vi "ROSServiceProvider.vi"(2 "Response":T2, 3 "ROS":T3={"topic port"=1236, "Node"="/labview", "topic"="/robot/head/command_head_nod", "type"="std_msgs/Bool", "node port"=7000, "error "={"status"=FALSE, "code"=0, "source"=""}, "Direction"=enum."Publisher", "Update (ms)"=1, "FIFO size"=1}) -> ()   [LabVIEW 2012]
doc: "Opens new ports for services, updates services with master, and closes services"
uses:
  Console/Servers/ServerSubs/MyState.ctl
  _ROSDefinition.vi
  MessageBuilding/std_msgs/subs/i16Scalar.vi
  MessageBuilding/std_msgs/subs/stringScalar.vi
  SubVIs/_ROSDirection.ctl
  SubVIs/_ROSControl.ctl
panel:
  out "Queue":string
  out "Master Reply":T1(array[cluster])
  out "response":string
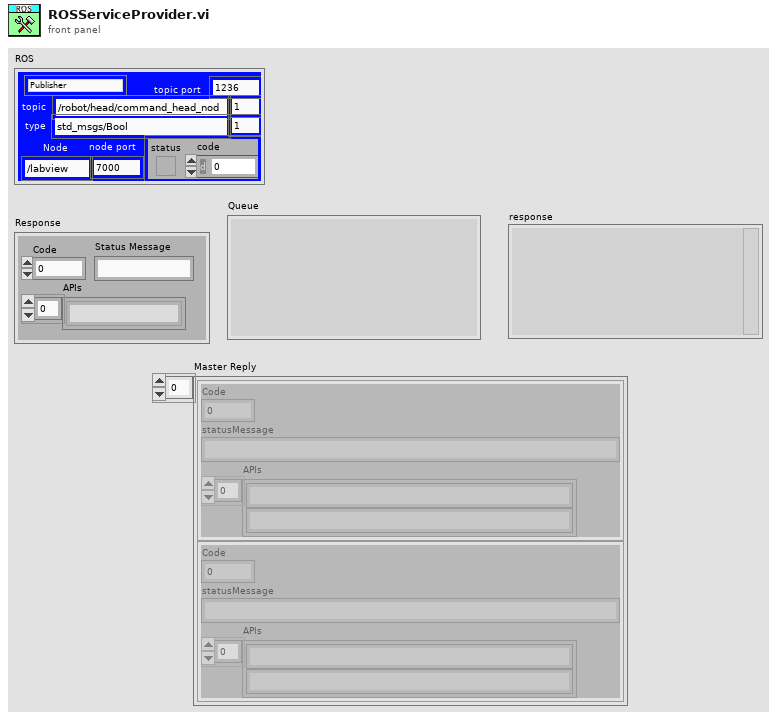
[diagram p1: front panel]
types:
  T1 = cluster{"Code":i8, "statusMessage":string, "APIs":string[]}[]
  T2 = cluster{"Code":i32, "Status Message":string, "APIs":string[]}
  T3 = typedef "_ROSControl.ctl" = cluster{"topic port":u16, "Node":string, "topic":string, "type":string, "node port":u16, "error ":errorcluster, "Direction":T4, "Update (ms)":u16, "FIFO size":u16}
  T4 = typedef "_ROSDirection.ctl" = enum16{"Node", "Publisher", "Subscriber", "ServiceClient", "ServiceProvider"}
  T5 = typedef "MyState.ctl" = enum16{"No Connection", "Registered", "Connected", "Close"}
  T6 = enum16{"Reset Log", "Add Client", "Remove Client", "Add Task"}
  T7 = typedef "ROSLog.ctl" = cluster{"Sent":string, "Reply":string, "MethodName":string, "success":bool, "Dir1":string, "Dir2":string, "Time Stamp":string, "error":errorcluster, "Preamble":string, "Midamble":string, "Postamble":string}
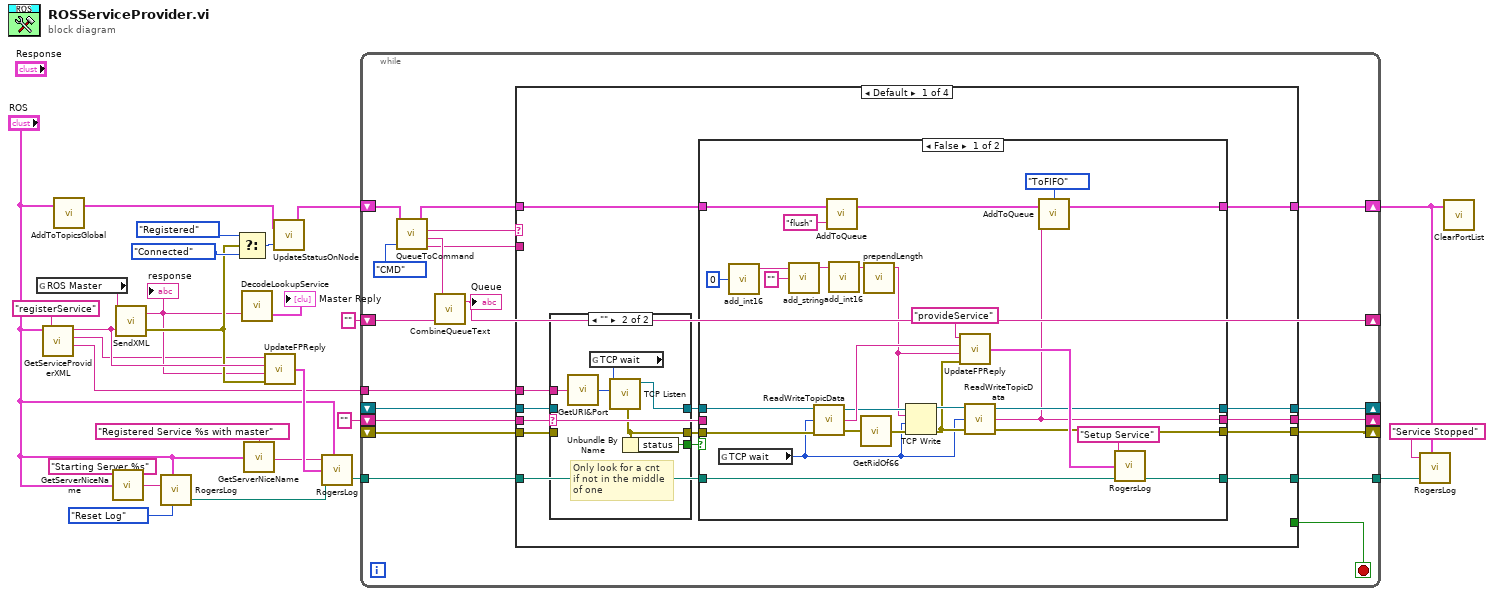
[diagram p0: block diagram]
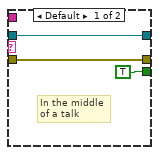
[diagram p2: hidden frame]
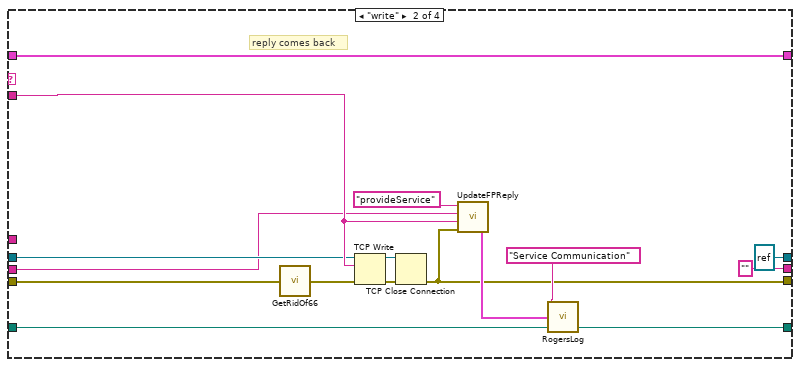
[diagram p4: hidden frame]
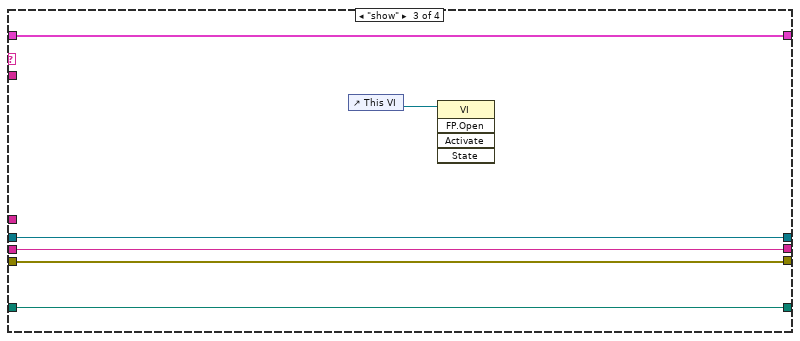
[diagram p5: hidden frame]
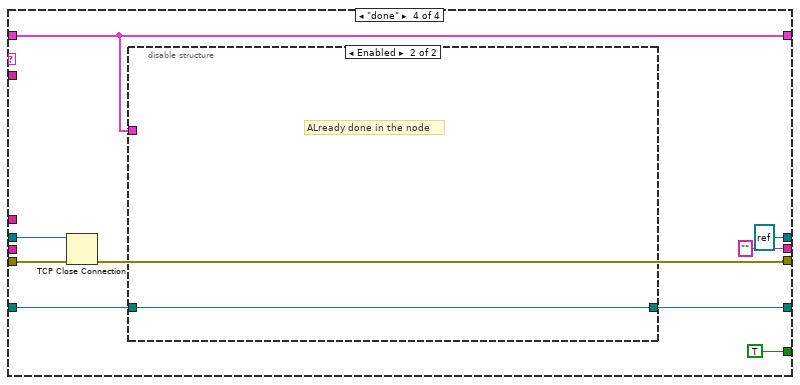
[diagram p6: hidden frame]
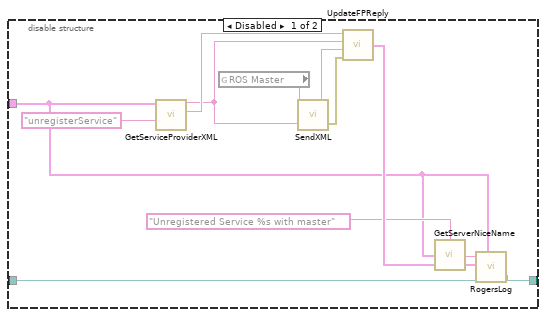
[diagram p7: hidden frame]
diagram:
  n1 = global read "_ROSDefinition.vi" "ROS Master"() -> (w23:string)
  n2 = call "GetServiceProviderXML.vi"("Method Name"="registerService", "ROS"="ROS") -> ("URI"=w6:string, "Method Name"=w9:string, "lookupService"=w24:string)  [unwired: 7 in]
  n3 = call "AddToTopicsGlobal.vi"("ROS in"="ROS") -> ("ROS out"=w3:T3)  [unwired: 2 in]
  n4 = call "GetServerNiceName.vi"("ROS"="ROS", "Text to add"="Starting Server %s") -> ("String"=w26:string)
  n5 = call "SendXML.vi"("Send"=w24, "URI in"=w23) -> ("error out"=w15:errorcluster, "Reply"=w14:string)
  "response" <- w14
  n6 = call "RogersLog.vi"("Text to add"=w26, "ROS"="ROS", "Task"=T6."Reset Log") -> ("LogPath out"=w18:path)  [unwired: 2 in, 1 out]
  n7 = Select(t=MyState."Registered" ("MyState"), s=w15, f=MyState."Connected" ("MyState")) -> (s? t:f=w20:T5)
  n8 = call "DecodeLookupService.vi"("Response"=w14) -> ("Reply"=→"Master Reply":T1)  [unwired: 2 in]
  n9 = call "GetServerNiceName.vi"("ROS"="ROS", "Text to add"="Registered Service %s with master") -> ("String"=w16:string)
  n10 = call "UpdateFPReply.vi"("error in (no error)"=w15, "Reply"=w14, "Sent"=w24, "method"=w9) -> ("Log"=w19:T7)
  n11 = call "UpdateStatusOnNode.vi"("MyState"=w20, "ROS"=w3) -> ("ROS out"=w2:T3)  [unwired: 1 in]
  n12 = call "RogersLog.vi"("Text to add"=w16, "ROS"="ROS", "Log"=w19, "LogPath in"=w18) -> ("LogPath out"=w11:path)  [unwired: 1 in, 1 out]
  n13 = while {
    tunnel: w11 -> [w46]
    tunnel: [w45] -> w10
    shift-right: [w41] -> _
    shift-left: "" ("New List") -> [w42]
    tunnel: w6 -> [w40]
    shift-right: [w35] -> _
    shift-left: _ -> [w32]
    shift-right: [w34] -> _
    shift-left: "" ("data out") -> [w30]
    shift-right: [w33] -> _
    shift-left: _ -> [w31]
    shift-right: [w28] -> w1
    shift-left: w2 -> [w39]
    stop <- w44 stop-if-true
    n14 = call "QueueToCommand.vi"("ROS"=w39, "Check"=enum16{"Cmd+FIFO", "FIFO", "CMD"}."CMD") -> ("ROS out"=w29:T3, "Command"=w37:string, "Queue log"=w43:string, "data"=w36:string)  [unwired: 1 in]
    n15 = call "CombineQueueText.vi"("Old List"=w42, "Queue In"=w43) -> ("New List"=w41:string)  [unwired: 1 in]
    "Queue" <- w41
    n16 = case shown="Default" w37 {
      tunnel: w29 -> [w59 w105 w123 w132]
      tunnel: w46 -> [w58 w108 w124 w131]
      tunnel: [w57 w107 w124 w130] -> w45
      tunnel: w36 -> [_ w113 _ _]
      tunnel: [w47 w105 w123 w132] -> w28
      tunnel: [_ _ _ TRUE] -> w44
      tunnel: w40 -> [w56 _ _ _]
      tunnel: [w55 refnum<k5> refnum ("connection ID out") w119 refnum<k5> refnum ("connection ID out")] -> w35
      tunnel: [w54 "" ("data out") w120 "" ("data out")] -> w34
      tunnel: [w53 w106 w121 w127] -> w33
      tunnel: w32 -> [w50 w111 w119 w128]
      tunnel: w31 -> [w51 w110 w121 w129]
      tunnel: w30 -> [w52 w109 w120 _]
      frame Default {
        n17 = case shown="\"\"" w52 {
          tunnel: [w63 w65] -> w49
          tunnel: [w62 w68] -> w60
          tunnel: w56 -> [_ w66]
          tunnel: w51 -> [w63 _]
          tunnel: w50 -> [w62 _]
          tunnel: [TRUE w64] -> w48
          frame Default {
            # "In the middle\nof a talk"
          }
          frame "" {
            # "Only look for a cnt\nif not in the middle\nof one"
            n18 = call "GetURI&Port.vi"("URI in"=w66) -> ("Port"=w69:u16)  [unwired: 1 out]
            n19 = global read "_ROSDefinition.vi" "TCP wait"() -> (w67:i32)
            n20 = call <vilib>:"TCP Listen.vi"("timeout ms (wait forever: -1)"=w67, "port"=w69) -> ("error out"=w65:errorcluster, "connection ID"=w68:refnum<k5>)  [unwired: 5 in, 3 out]
            n21 = Unbundle By Name(w65) -> ("status"=w64:bool)
          }
        }
        n22 = case shown="False" w48 {
          tunnel: w60 -> [w97 w101]
          tunnel: w58 -> [w93 w102]
          tunnel: w59 -> [w72 w98]
          tunnel: [w76 w102] -> w57
          tunnel: [w79 w101] -> w55
          tunnel: [w78 w100] -> w54
          tunnel: [w77 w99] -> w53
          tunnel: w52 -> [_ w100]
          tunnel: w49 -> [w75 w99]
          tunnel: [w70 w98] -> w47
          frame False {
            n23 = global read "_ROSDefinition.vi" "TCP wait"() -> (w74:i32)
            n24 = call-poly "add_int16.vi"("Numeric"=i16 0) -> ("msg out"=w89:string)  [unwired: 4 in]
            n25 = call-poly "add_string.vi"("String"="", "msg in"=w89) -> ("msg out"=w90:string)  [unwired: 3 in]
            n26 = call "ReadWriteTopicData.vi"("error in (no error)"=w75, "timeout ms (1000)"=w74, "connection ID in"=w97) -> ("error out"=w96:errorcluster, "data out"=w95:string, "connection ID out"=w87:refnum<k5>)
            n27 = call "AddToQueue.vi"("Cmd"="flush", "ROS"=w72) -> ("ROS out"=w71:T3)  [unwired: 3 in]
            n28 = call-poly "add_int16.vi"("msg in"=w90) -> ("msg out"=w82:string)  [unwired: 4 in]
            n29 = call "GetRidOf66.vi"("error in (no error)"=w96) -> ("error out"=w88:errorcluster)
            n30 = call "prependLength.vi"("msg in"=w82) -> ("msg out"=w81:string)  [unwired: 4 in]
            n31 = TCP Write(connection ID=w87, data in=w81, error in (no error)=w88, 9:w74) -> (connection ID out=w86:refnum<k5>, error out=w85:errorcluster)  [unwired: 1 out]
            n32 = call "UpdateFPReply.vi"("error in (no error)"=w85, "Reply"=w81, "Sent"=w95, "method"="provideService") -> ("Log"=w84:T7)
            n33 = call "ReadWriteTopicData.vi"("error in (no error)"=w85, "timeout ms (1000)"=w74, "connection ID in"=w86) -> ("error out"=w77:errorcluster, "data out"=w78:string, "connection ID out"=w79:refnum<k5>)
            n34 = call "AddToQueue.vi"("Cmd"=w78, "ROS"=w71, "Type"=enum16{"topic", "node", "ToFIFO"}."ToFIFO") -> ("ROS out"=w70:T3)  [unwired: 2 in]
            n35 = call "RogersLog.vi"("Text to add"="Setup Service", "Log"=w84, "LogPath in"=w93) -> ("LogPath out"=w76:path)  [unwired: 2 in, 1 out]
          }
          frame True {
          }
        }
      }
      frame "write" {
        # "reply comes back"
        n36 = call "GetRidOf66.vi"("error in (no error)"=w110) -> ("error out"=w118:errorcluster)
        n37 = TCP Write(connection ID=w111, data in=w113, error in (no error)=w118) -> (connection ID out=w116:refnum<k5>, error out=w117:errorcluster)  [unwired: 1 in, 1 out]
        n38 = TCP Close Connection(connection ID=w116, error in (no error)=w117) -> (error out=w106:errorcluster)  [unwired: 1 in, 1 out]
        n39 = call "UpdateFPReply.vi"("error in (no error)"=w106, "Reply"=w113, "Sent"=w109, "method"="provideService") -> ("Log"=w114:T7)
        n40 = call "RogersLog.vi"("Text to add"="Service Communication", "Log"=w114, "LogPath in"=w108) -> ("LogPath out"=w107:path)  [unwired: 2 in, 1 out]
      }
      frame "show" {
        n41 = control-ref of="This VI"() -> (w122:refnum<vi>)
        n42 = invoke class="VI" method="FP.Open"(reference=w122) -> ()  [unwired: 4 in, 5 out]
      }
      frame "done" {
        n43 = TCP Close Connection(connection ID=w128, error in (no error)=w129) -> (error out=w127:errorcluster)  [unwired: 1 in, 1 out]
        n44 = disable-structure shown="Enabled" {
          disable-tunnel: w132 -> [w137 _]
          disable-tunnel: w131 -> [w135 w146]
          disable-tunnel: [w134 w146] -> w130
          frame Disabled {
            n45 = call "GetServiceProviderXML.vi"("Method Name"="unregisterService", "ROS"=w137) -> ("Method Name"=w142:string, "lookupService"=w141:string)  [unwired: 7 in, 1 out]
            n46 = global read "_ROSDefinition.vi" "ROS Master"() -> (w145:string)
            n47 = call "SendXML.vi"("Send"=w141, "URI in"=w145) -> ("error out"=w143:errorcluster, "Reply"=w140:string)
            n48 = call "UpdateFPReply.vi"("error in (no error)"=w143, "Reply"=w140, "Sent"=w141, "method"=w142) -> ("Log"=w139:T7)
            n49 = call "GetServerNiceName.vi"("ROS"=w137, "Text to add"="Unregistered Service %s with master") -> ("String"=w136:string)
            n50 = call "RogersLog.vi"("Text to add"=w136, "ROS"=w137, "Log"=w139, "LogPath in"=w135) -> ("LogPath out"=w134:path)  [unwired: 1 in, 1 out]
          }
          frame Enabled {
            # "ALready done in the node"
          }
        }
      }
    }
  }
  n51 = call "RogersLog.vi"("Text to add"="Service Stopped", "ROS"=w1, "LogPath in"=w10) -> ()  [unwired: 2 in, 2 out]
  n52 = call "ClearPortList.vi"("ROS"=w1) -> ()  [unwired: 2 in]
